vi "_CSMObj-Generate Worker Agent.vi"(8 "Error in":errorcluster caption="Error in (no error)", 11 "CSMObj in":T1) -> (0 "Error out":errorcluster, 2 "Agent":T1, 3 "CSMObj out":T1)   [LabVIEW 2014, in "Communicable State Machine.lvlib"]
uses:
  Communicable State Machine.lvlib
  _CSMObj.ctl
  Priority Queue/Priority Queue.lvclass
  Typedef/_CSM_MODE.ctl
  _CSMObj-Data.ctl
  Typedef/_CSM Status Change Event Data.ctl
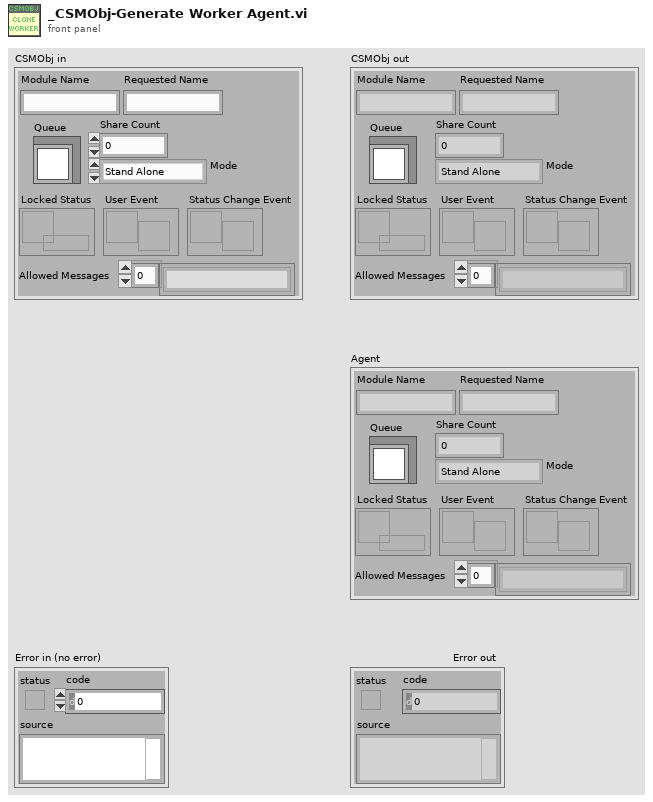
[diagram p1: front panel]
types:
  T1 = typedef "Communicable State Machine.lvlib/_CSMObj.ctl" = cluster{"Requested Name":string, "Module Name":string, "Mode":T2, "Share Count":i32, "Queue":refnum<class "Priority Queue.lvclass">, "Locked Status":refnum<data-value>, "User Event":refnum<user-event>, "Status Change Event":refnum<user-event>, "Allowed Messages":string[]}
  T2 = typedef "Communicable State Machine.lvlib/_CSM_MODE.ctl" = enum16{"Stand Alone", "CSM", "Worker Agent", "Action Worker", "Chain", "Chain Node"}
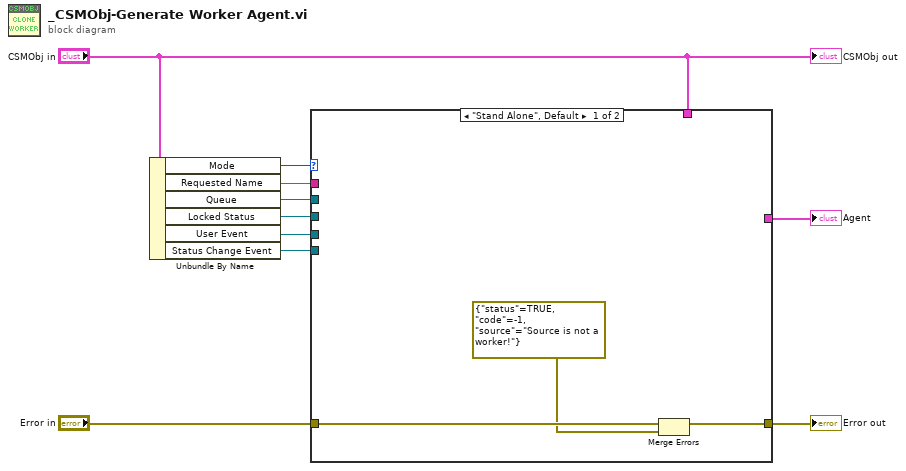
[diagram p0: block diagram]
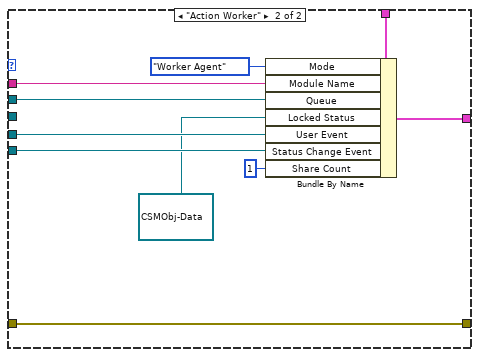
[diagram p2: hidden frame]
diagram:
  n1 = Unbundle By Name("CSMObj in") -> ("Mode"=w6:T2, "Requested Name"=w9:string, "Queue"=w8:refnum<class "Priority Queue.lvclass">, "Locked Status"=w1:refnum<data-value>, "User Event"=w2:refnum<user-event>, "Status Change Event"=w3:refnum<user-event>)
  n2 = case shown="\"Stand Alone\", Default" w6 {
    tunnel: "CSMObj in" -> [_ w22]
    tunnel: w9 -> [_ w21]
    tunnel: w8 -> [_ w20]
    tunnel: [_ w19] -> w7
    tunnel: "Error in" -> [w13 w18]
    tunnel: [w12 w18] -> w4
    tunnel: w3 -> [_ w16]
    tunnel: w2 -> [_ w15]
    tunnel: w1 -> [_ _]
    frame "Stand Alone", Default {
      n3 = Merge Errors(w13, errorcluster {"status"=TRUE, "code"=-1, "source"="Source is not a worker!"} ("error in")) -> (w12:errorcluster)
    }
    frame "Action Worker" {
      n4 = Bundle By Name(cluster=w22, "Mode"=_CSM_MODE."Worker Agent", "Module Name"=w21, "Queue"=w20, "Locked Status"=refnum<data-value> refnum, "User Event"=w15, "Status Change Event"=w16, "Share Count"=1) -> (w19:T1)
    }
  }
  "Error out" <- w4
  "Agent" <- w7
  "CSMObj out" <- "CSMObj in"
